vi "WSVCAP SHL Host LL Build Top Level FPGA VI Path.vi"(11 "Error In (no error)":errorcluster) -> (4 "Top Level FPGA VI Path":path, 15 "Error Out":errorcluster)   [LabVIEW 2012]
panel:
  out "Top Level Host VI Directory":path
  out "Development Environment":bool
  out "Top Level FPGA VI Directory":path
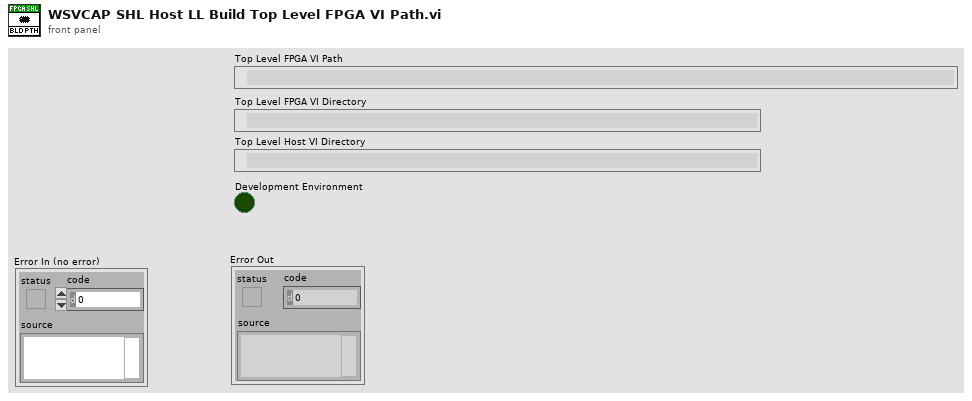
[diagram p1: front panel]
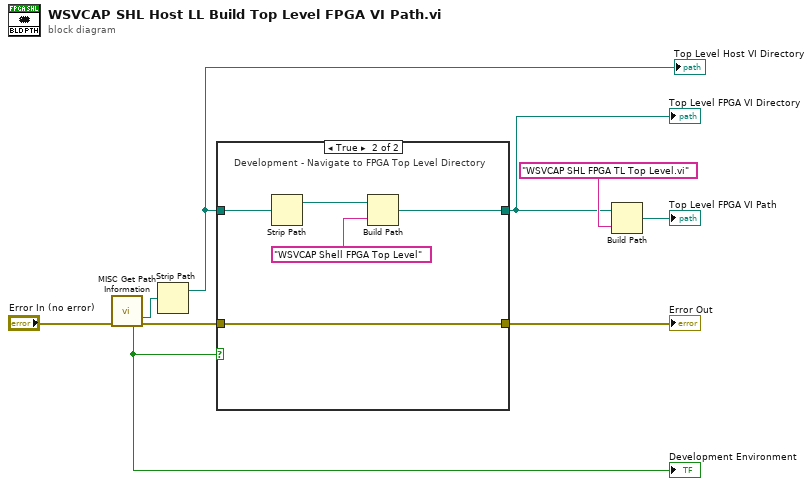
[diagram p0: block diagram]
diagram:
  n1 = call "MISC Get Path Information.vi"("Error In (no error)"="Error In (no error)") -> ("Top Level VI Path"=w9:path, "Development Environment"=w7:bool, "Error Out"=w6:errorcluster)  [unwired: 8 in, 4 out]
  "Development Environment" <- w7
  n2 = Strip Path(path=w9) -> (stripped path=w1:path)  [unwired: 1 out]
  "Top Level Host VI Directory" <- w1
  n3 = case shown="True" w7 {
    tunnel: w1 -> [w10 w15]
    tunnel: [w10 w13] -> w3
    tunnel: [w11 w16] -> w5
    tunnel: w6 -> [w11 w16]
    frame False {
      # "Executable - All VIs at same level in hierarchy (.exe)"
    }
    frame True {
      # "Development - Navigate to FPGA Top Level Directory"
      n4 = Strip Path(path=w15) -> (stripped path=w14:path)  [unwired: 1 out]
      n5 = Build Path(base path=w14, name or relative path="WSVCAP Shell FPGA Top Level") -> (appended path=w13:path)
    }
  }
  "Error Out" <- w5
  "Top Level FPGA VI Directory" <- w3
  n6 = Build Path(base path=w3, name or relative path="WSVCAP SHL FPGA TL Top Level.vi") -> (appended path=→"Top Level FPGA VI Path":path)
